vi "EMV Sample History.vi"(8 "error in (no error)":errorcluster, 10 "length":i32=10, 11 "T6 Temp":dbl) -> (0 "error out":errorcluster, 3 "T6 History":dbl[](array[numeric]))   [LabVIEW 2016]
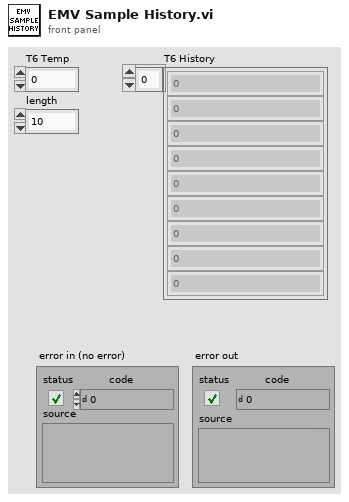
[diagram p1: front panel]
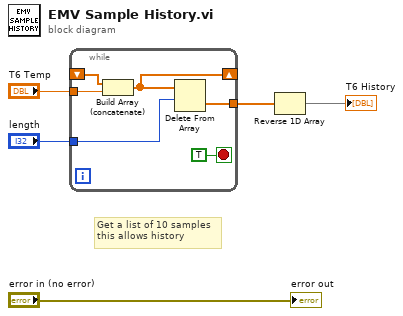
[diagram p0: block diagram]
diagram:
  # "Get a list of 10 samples \nthis allows history"
  n1 = while {
    shift-right: [w10] -> _
    shift-left: _ -> [w11]
    tunnel: "T6 Temp" -> [w8]
    tunnel: [w7] -> w3
    tunnel: "length" -> [w6]
    stop <- TRUE stop-if-true
    n2 = Build Array (concatenate)(w11, w8) -> (w10:dbl[])
    n3 = Delete From Array(array=w10, length=w6) -> (deleted portion=w7:dbl[])  [unwired: 1 in, 1 out]
  }
  n4 = Reverse 1D Array(array=w3) -> (reversed array=→"T6 History":dbl[])
  "error out" <- "error in (no error)"
